vi "Error Check Transform.vi"(8 "error in (no error)":errorcluster, 11 "Transform in":T1) -> (0 "error out":errorcluster, 3 "Transform out":T1)   [LabVIEW 2017, in "NI_Kinematics.lvlib"]
uses:
  <vilib>/robotics/Kinematics/NI_Kinematics.lvlib
  <vilib>/Analysis/Matrix/Datatypes/RealMatrix.ctl
  <vilib>/robotics/Utilities/NI_Robotics Utilities.lvlib
  <vilib>/Analysis/Matrix/NI_Matrix.lvlib
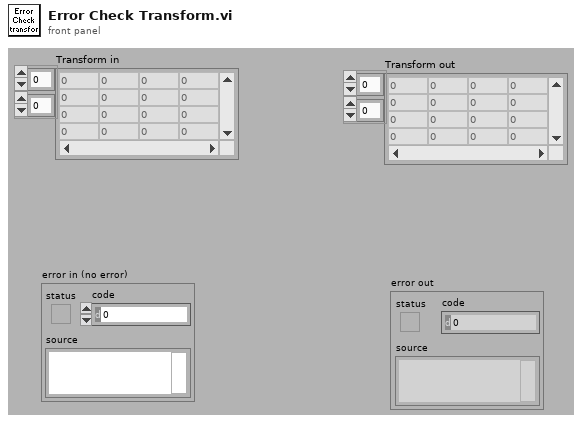
[diagram p1: front panel]
types:
  T1 = typedef "NI_Matrix.lvlib/RealMatrix.ctl" = dbl[][]
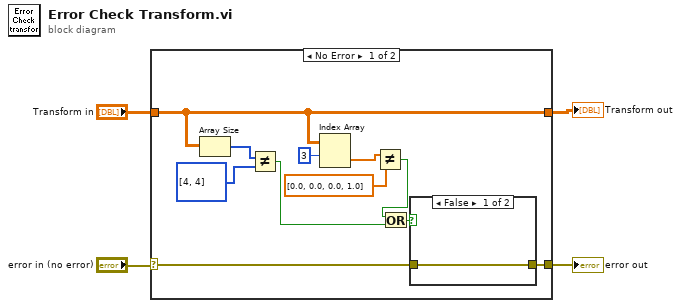
[diagram p0: block diagram]
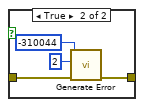
[diagram p2: hidden frame]
diagram:
  n1 = case shown="No Error" "error in (no error)" {
    selector: "error in (no error)" -> [w6 w21]
    tunnel: "Transform in" -> [w13 w22]
    tunnel: [w13 w22] -> w2
    tunnel: [w5 w21] -> w1
    frame No Error {
      n2 = Array Size(array=w13) -> (size(s)=w15:i32[])
      n3 = Not Equal?(x=w15, y=i32[] [4, 4] ("size(s)")) -> (x != y?=w7:bool)
      n4 = Index Array(array=w13, index (row)=3) -> (element=w11:dbl[])  [unwired: 1 in]
      n5 = Not Equal?(x=w11, y=dbl[] [0.0, 0.0, 0.0, 1.0] ("subarray")) -> (x != y?=w8:bool)
      n6 = Or(x=w8, y=w7) -> (x .or. y?=w9:bool)
      n7 = case shown="False" w9 {
        tunnel: w6 -> [w16 w20]
        tunnel: [w16 w19] -> w5
        frame False {
        }
        frame True {
          n8 = call <vilib>:"Generate Error.vi"("error in (no error)"=w20, "chain levels to remove (1)"=2, "code"=-310044) -> ("error out"=w19:errorcluster)  [unwired: 8 in]
        }
      }
    }
    frame Error {
    }
  }
  "error out" <- w1
  "Transform out" <- w2
